vi "Subvi photocounter.vi"(5 "DIchannel":refnum<k21>="Connector0/DIO1", 11 "Reset":bool) -> (1 "PMTmon":bool, 2 "PMTedgeChangeMon":bool, 6 "Count":u8)   [LabVIEW 2017]
uses:
  <vilib>/rvi/eio/common/nirviEmuTemplateMethod_errors.vi
  <vilib>/eio/EIONode/EIONode.xnode
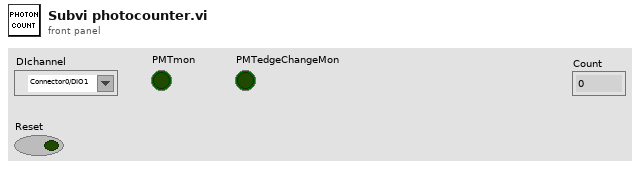
[diagram p1: front panel]
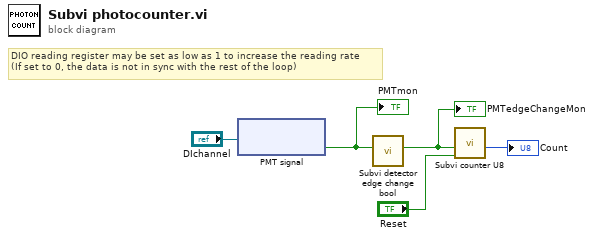
[diagram p0: block diagram]
diagram:
  # "DIO reading register may be set as low as 1 to increase the reading rate\n(If set to 0, the data is not in sync with the rest of the loop)"
  n1 = xnode "PMT signal"("FPGA I/O In"="DIchannel") -> ("I/O Item"=w4:bool)  [unwired: 1 out]
  "PMTmon" <- w4
  n2 = call "Subvi detector edge change bool.vi"("Input"=w4) -> ("Output"=w1:bool)  [unwired: 8 in]
  "PMTedgeChangeMon" <- w1
  n3 = call "Subvi counter U8.vi"("Reset"="Reset", "+1"=w1) -> ("Count"=→"Count":u8)  [unwired: 9 in]
